vi "Revision Query.vi"(8 "error in (no error)":errorcluster, 11 "VISA resource name":refnum<visa-resource-name>) -> (0 "error out":errorcluster, 1 "Driver Revision":string, 2 "Firmware Revision":string, 3 "VISA resource name out":refnum<visa-resource-name>)   [LabVIEW 2009, in "Digikrom DK24x.lvlib"]
doc: "Queries the current instrument firmware revision and instrument driver revision.\n\nRefer to the Readme file for detailed driver information including modification history."
uses:
  Digikrom DK24x.lvlib
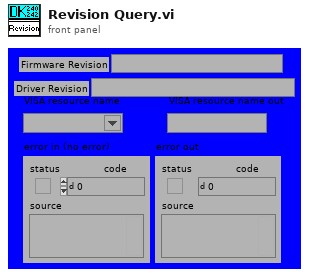
[diagram p1: front panel]
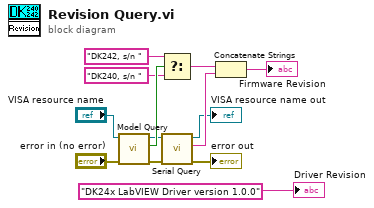
[diagram p0: block diagram]
diagram:
  n1 = call "Model Query.vi"("error in (no error)"="error in (no error)", "VISA resource name"="VISA resource name") -> ("error out"=w5:errorcluster, "Is DK242?"=w11:bool, "VISA resource name out"=w6:refnum<visa-resource-name>)  [unwired: 7 out]
  n2 = Select(t="DK242, s/n ", s=w11, f="DK240, s/n ") -> (s? t:f=w8:string)
  n3 = call "Serial Query.vi"("error in (no error)"=w5, "VISA resource name"=w6) -> ("error out"=→"error out":errorcluster, "SERIAL"=w7:string, "VISA resource name out"=→"VISA resource name out":refnum<visa-resource-name>)  [unwired: 7 out]
  n4 = Concatenate Strings(w8, w7) -> (→"Firmware Revision":string)
  "Driver Revision" <- "DK24x LabVIEW Driver version 1.0.0"
